vi "cor_regressao.vi"() -> ()   [LabVIEW 2016]
uses:
  <vilib>/NXT/Subs/LVHSConnector.ctl
  <vilib>/NXT/LegoClasses/BrickReference/BrickReference.lvclass
  <vilib>/NXT/Subs/ColorSensorColors.ctl
  <vilib>/NXT/Block Support/NXT_InputPort.ctl
panel:
  out "Detected Color":T1=enum."Green"
  out "NXT/EV3 3":T2
  in  "NXT/EV3 2":T2
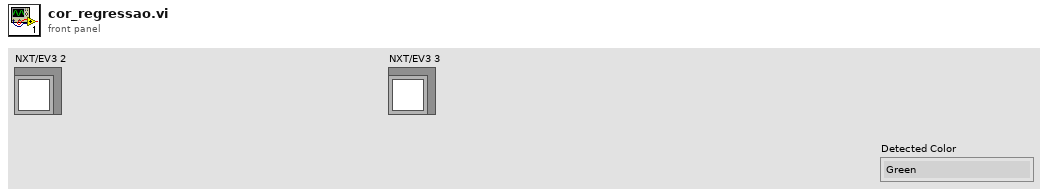
[diagram p1: front panel]
types:
  T1 = typedef "ColorSensorColors.ctl" = enum16{"No Color", "Black", "Blue", "Green", "Yellow", "Red", "White", "Brown"}
  T2 = typedef "LVHSConnector.ctl" = refnum<class "BrickReference.lvclass">
  T3 = typedef "NXT_InputPort.ctl" = u32
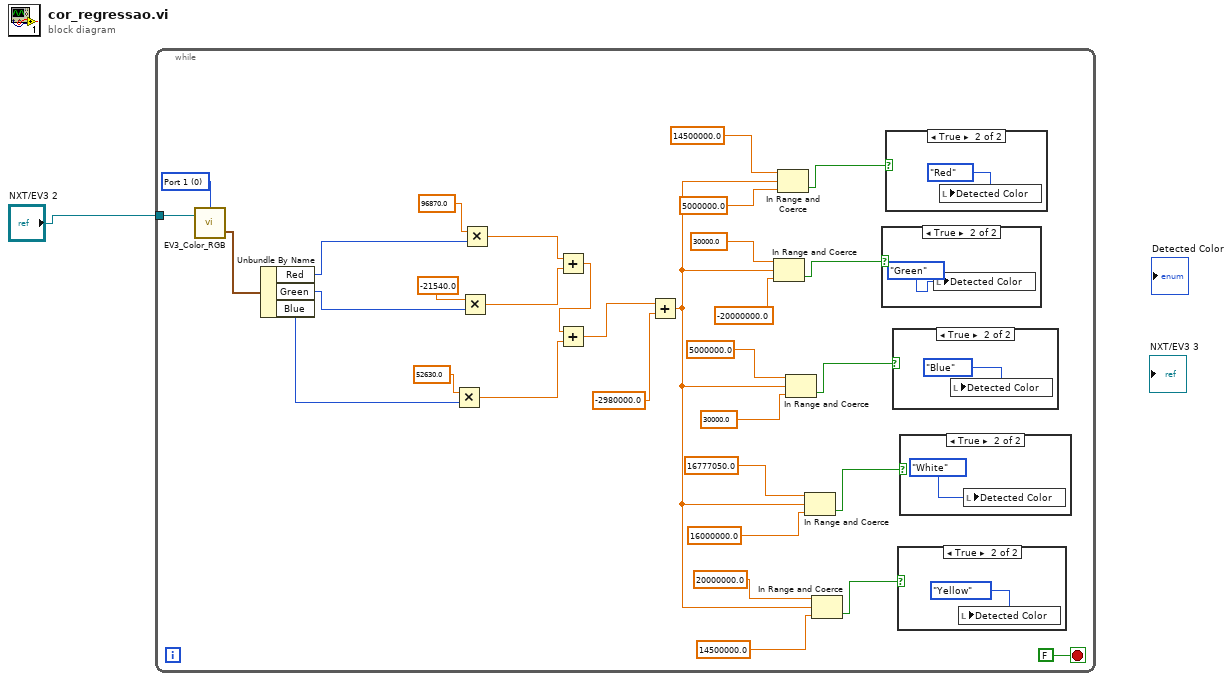
[diagram p0: block diagram]
diagram:
  n1 = while {
    tunnel: "NXT/EV3 2" -> [w33]
    stop <- FALSE stop-if-true
    w2 = T3 0 items=["Port 1", "Port 2", "Port 3", "Port 4"] ("Port (Port 1)")
    n2 = call <vilib>:"EV3_Color_RGB.vi"("NXT/EV3"=w33, "Port (Port 1)"=w2) -> ("RGB Color"=w32:cluster{"Red":u8, "Green":u8, "Blue":u8})  [unwired: 1 in, 1 out]
    n3 = Unbundle By Name(w32) -> ("Red"=w6:u8, "Green"=w5:u8, "Blue"=w4:u8)
    n4 = Multiply(x=52630.0, y=w4) -> (x*y=w9:dbl)
    n5 = Multiply(x=-21540.0, y=w5) -> (x*y=w11:dbl)
    n6 = Multiply(x=96870.0, y=w6) -> (x*y=w12:dbl)
    n7 = Add(x=w12, y=w11) -> (x+y=w10:dbl)
    n8 = Add(x=w10, y=w9) -> (x+y=w8:dbl)
    n9 = Add(x=w8, y=-2980000.0) -> (x+y=w21:dbl)
    n10 = In Range and Coerce(upper limit=30000.0, x=w21, lower limit=-20000000.0) -> (In Range?=w19:bool)  [unwired: 1 out]
    n11 = In Range and Coerce(upper limit=14500000.0, x=w21, lower limit=5000000.0) -> (In Range?=w20:bool)  [unwired: 1 out]
    n12 = In Range and Coerce(upper limit=5000000.0, x=w21, lower limit=30000.0) -> (In Range?=w18:bool)  [unwired: 1 out]
    n13 = In Range and Coerce(upper limit=16777050.0, x=w21, lower limit=16000000.0) -> (In Range?=w17:bool)  [unwired: 1 out]
    n14 = In Range and Coerce(upper limit=20000000.0, x=w21, lower limit=14500000.0) -> (In Range?=w16:bool)  [unwired: 1 out]
    n15 = case shown="True" w19 {
      frame False {
      }
      frame True {
        n16 = local write "Detected Color"(ColorSensorColors."Green" ("Detected Color")) -> ()
      }
    }
    n17 = case shown="True" w20 {
      frame False {
      }
      frame True {
        n18 = local write "Detected Color"(ColorSensorColors."Red" ("Detected Color")) -> ()
      }
    }
    n19 = case shown="True" w18 {
      frame False {
      }
      frame True {
        n20 = local write "Detected Color"(ColorSensorColors."Blue" ("Detected Color")) -> ()
      }
    }
    n21 = case shown="True" w16 {
      frame False {
      }
      frame True {
        n22 = local write "Detected Color"(ColorSensorColors."Yellow" ("Detected Color")) -> ()
      }
    }
    n23 = case shown="True" w17 {
      frame False {
      }
      frame True {
        n24 = local write "Detected Color"(ColorSensorColors."White" ("Detected Color")) -> ()
      }
    }
  }
